vi "ini配置文件写入（U32）.vi"(8 "value":u32 caption="值", 9 "key":string="调色板阶数", 10 "section":string="系统", 11 "文件名称":string="配置文件") -> ()   [LabVIEW 2018]
uses:
  <vilib>/Utility/error.llb/DialogType.ctl
  <vilib>/Utility/config.llb/Write Key (U32).vi
  <vilib>/Utility/config.llb/NI_LVConfig.lvlib
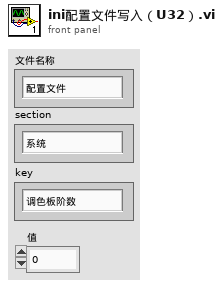
[diagram p1: front panel]
types:
  T1 = typedef "DialogType.ctl" = u16
  T2 = typedef "NI_LVConfig.lvlib/Config Data RefNum.ctl" = refnum<k1>
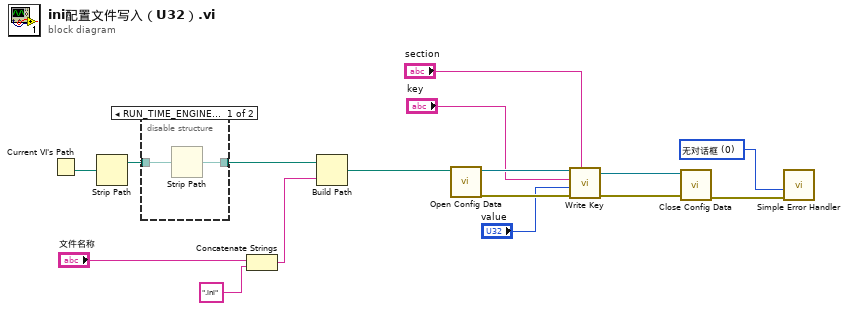
[diagram p0: block diagram]
diagram:
  w4 = T1 0 items=["无对话框", "确定信息", "继续或停止信息", "确定信息＋警告", "继续/停止+警告"] ("type of dialog (OK msg:1)")
  n1 = Current VI's Path() -> (path=w11:path)
  n2 = Strip Path(path=w11) -> (stripped path=w10:path)  [unwired: 1 out]
  n3 = disable-structure shown="RUN_TIME_ENGINE==True" {
    disable-tunnel: w10 -> [w18 w19]
    disable-tunnel: [w17 w19] -> w9
    frame condition #0 {
      n4 = Strip Path(path=w18) -> (stripped path=w17:path)  [unwired: 1 out]
    }
    frame condition #1 (active) {
    }
  }
  n5 = Concatenate Strings("文件名称", ".ini" ("字符串")) -> (w7:string)
  n6 = Build Path(base path=w9, name or relative path=w7) -> (appended path=w16:path)
  n7 = call <vilib>:"Open Config Data.vi"("configuration file path"=w16) -> ("error out"=w2:errorcluster, "refnum"=w15:T2)  [unwired: 2 in, 7 out]
  n8 = call-poly <vilib>:"Write Key.vi"("section"="section", "error in (no error)"=w2, "value"="value", "key"="key", "refnum"=w15) -> ("error out"=w3:errorcluster, "refnum out"=w12:T2)  [unwired: 4 in, 1 out]
  n9 = call <vilib>:"Close Config Data.vi"("error in (no error)"=w3, "refnum"=w12) -> ("error out"=w5:errorcluster)  [unwired: 1 in, 8 out]
  n10 = call <vilib>:"Simple Error Handler.vi"("type of dialog (OK msg:1)"=w4, "error in (no error)"=w5) -> ()  [unwired: 8 out]
